vi "P4CMD Dialog_SetCtlDisableProp.vi"(7 "P4Proj UIDialog FP Refs":T1, 8 "error in (no error)":errorcluster, 10 "use defaults?":bool) -> (0 "error out":errorcluster)   [LabVIEW 2017, in "NI_SCC_P4CMD.lvlib"]
uses:
  <vilib>/SourceControl/Providers/P4CMD/NI_SCC_P4CMD.lvlib
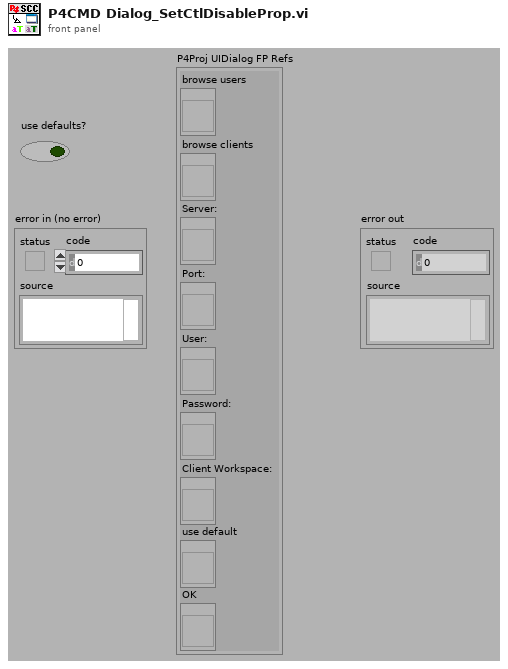
[diagram p1: front panel]
types:
  T1 = cluster{"browse users":refnum<vi>, "browse clients":refnum<vi>, "Server:":refnum<vi>, "Port:":refnum<vi>, "User:":refnum<vi>, "Password:":refnum<vi>, "Client Workspace:":refnum<vi>, "use default":refnum<vi>, "OK":refnum<vi>}
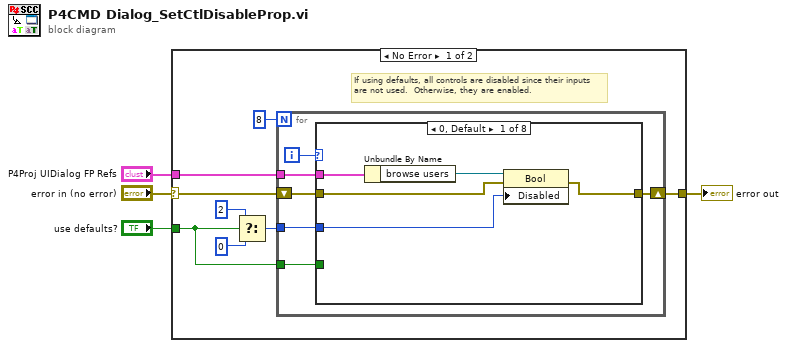
[diagram p0: block diagram]
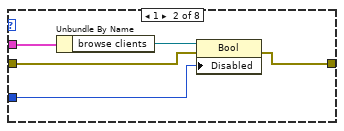
[diagram p2: hidden frame]
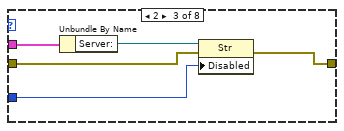
[diagram p3: hidden frame]
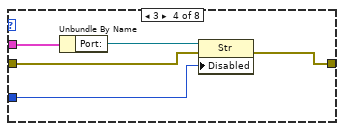
[diagram p4: hidden frame]
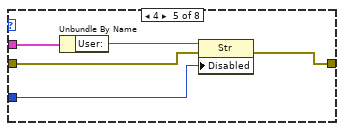
[diagram p5: hidden frame]
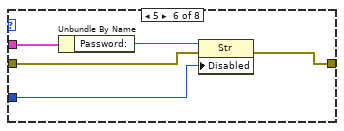
[diagram p6: hidden frame]
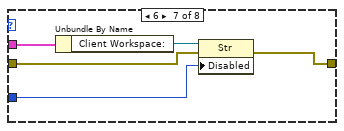
[diagram p7: hidden frame]
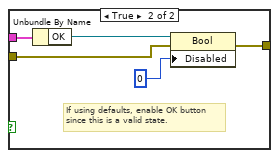
[diagram p9: hidden frame]
diagram:
  n1 = case shown="No Error" "error in (no error)" {
    selector: "error in (no error)" -> [w6 w64]
    tunnel: "P4Proj UIDialog FP Refs" -> [w7 _]
    tunnel: [w9 w64] -> w3
    tunnel: "use defaults?" -> [w5 _]
    frame No Error {
      # "If using defaults, all controls are disabled since their inputs are not used.  Otherwise, they are enabled."
      n2 = Select(t=u8 2 ("Disabled"), s=w5, f=u8 0) -> (s? t:f=w8:u8)
      n3 = for {
        N: 8 -> [_]
        tunnel: w7 -> [w18]
        tunnel: w8 -> [w14]
        shift-right: [w15] -> w9
        shift-left: w6 -> [w16]
        tunnel: w5 -> [w13]
        i -> [w17]
        n4 = case shown="0, Default" w17 {
          tunnel: w18 -> [w23 w28 w33 w38 w43 w48 w53 w57]
          tunnel: w16 -> [w21 w26 w31 w36 w41 w46 w51 w56]
          tunnel: w14 -> [w20 w25 w30 w35 w40 w45 w50 _]
          tunnel: [w19 w24 w29 w34 w39 w44 w49 w55] -> w15
          tunnel: w13 -> [_ _ _ _ _ _ _ w54]
          frame 0, Default {
            n5 = Unbundle By Name(w23) -> ("browse users"=w22:refnum<vi>)
            n6 = property class="Bool"(reference=w22, error in=w21, "Disabled"=w20) -> (error out=w19:errorcluster)  [unwired: 1 out]
          }
          frame 1 {
            n7 = Unbundle By Name(w28) -> ("browse clients"=w27:refnum<vi>)
            n8 = property class="Bool"(reference=w27, error in=w26, "Disabled"=w25) -> (error out=w24:errorcluster)  [unwired: 1 out]
          }
          frame 2 {
            n9 = Unbundle By Name(w33) -> ("Server:"=w32:refnum<vi>)
            n10 = property class="Str"(reference=w32, error in=w31, "Disabled"=w30) -> (error out=w29:errorcluster)  [unwired: 1 out]
          }
          frame 3 {
            n11 = Unbundle By Name(w38) -> ("Port:"=w37:refnum<vi>)
            n12 = property class="Str"(reference=w37, error in=w36, "Disabled"=w35) -> (error out=w34:errorcluster)  [unwired: 1 out]
          }
          frame 4 {
            n13 = Unbundle By Name(w43) -> ("User:"=w42:refnum<vi>)
            n14 = property class="Str"(reference=w42, error in=w41, "Disabled"=w40) -> (error out=w39:errorcluster)  [unwired: 1 out]
          }
          frame 5 {
            n15 = Unbundle By Name(w48) -> ("Password:"=w47:refnum<vi>)
            n16 = property class="Str"(reference=w47, error in=w46, "Disabled"=w45) -> (error out=w44:errorcluster)  [unwired: 1 out]
          }
          frame 6 {
            n17 = Unbundle By Name(w53) -> ("Client Workspace:"=w52:refnum<vi>)
            n18 = property class="Str"(reference=w52, error in=w51, "Disabled"=w50) -> (error out=w49:errorcluster)  [unwired: 1 out]
          }
          frame 7 {
            n19 = case shown="False" w54 {
              tunnel: w57 -> [_ w63]
              tunnel: w56 -> [w58 w61]
              tunnel: [w58 w60] -> w55
              frame False {
              }
              frame True {
                # "If using defaults, enable OK button since this is a valid state."
                n20 = Unbundle By Name(w63) -> ("OK"=w62:refnum<vi>)
                n21 = property class="Bool"(reference=w62, error in=w61, "Disabled"=u8 0) -> (error out=w60:errorcluster)  [unwired: 1 out]
              }
            }
          }
        }
      }
    }
    frame Error {
    }
  }
  "error out" <- w3
